vi "pitcherSpike.vi"   [LabVIEW 2011]
types:
  T1 = typedef "WPI_RelayDevRef.ctl" = cluster{"DevStatus":errorcluster, "Relay Channel":T2, "Digital Module":T3, "Relay Direction":T4}
  T2 = typedef "FPGA_DIORelayChannel.ctl" = enum8{"Relay 1", "Relay 2", "Relay 3", "Relay 4", "Relay 5", "Relay 6", "Relay 7", "Relay 8", "Invalid"}
  T3 = typedef "FPGA_TypedefDigitalModule.ctl" = enum16{"Digital Module 1", "Digital Module 2"}
  T4 = typedef "WPI_RelayDirection.ctl" = enum16{"Both directions", "Forward only", "Reverse only"}
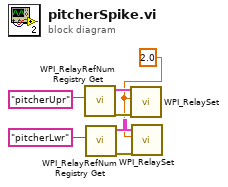
[diagram p0: block diagram]
diagram:
  w1 = 2.0 ("Output")
  n1 = call <vilib>:"WPI_RelayRefNum Registry Get.vi"("refnum name"="pitcherUpr") -> ("error out"=w3:errorcluster, "RelayDevRef"=w4:T1)  [unwired: 9 in]
  n2 = call <vilib>:"WPI_RelayRefNum Registry Get.vi"("refnum name"="pitcherLwr") -> ("error out"=w2:errorcluster, "RelayDevRef"=w5:T1)  [unwired: 9 in]
  n3 = call <vilib>:"WPI_RelaySet.vi"("error in (no error)"=w3, "RelayValue"=w1, "RelayDevRef"=w4) -> ()  [unwired: 7 in, 2 out]
  n4 = call <vilib>:"WPI_RelaySet.vi"("error in (no error)"=w2, "RelayValue"=w1, "RelayDevRef"=w5) -> ()  [unwired: 7 in, 2 out]
